vi "Destroy.vi"(0 "reference":refnum<class "CallNode.lvclass">, 5 "error in (no error)":errorcluster) -> (15 "# of objects":i32, 19 "error out":errorcluster)   [LabVIEW 2014, in "CallNode.lvclass"]
doc: "Destroys a CallNode object created with a CallNode constructor VI.\n\n[GOOP 2.3]"
uses:
  <resource>/Framework/Providers/Open_GDS/UML/CallNode_class/CallNode.lvclass
  <resource>/Framework/Providers/Open_GDS/UML/RectangularNode_class/RectangularNode.lvclass
panel:
  out "reference out":refnum<class "CallNode.lvclass">
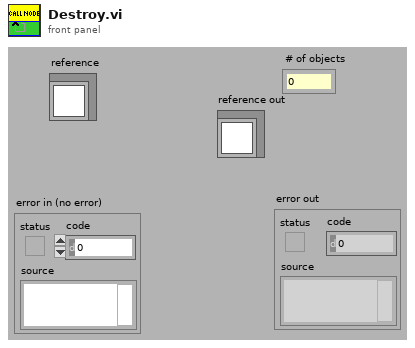
[diagram p1: front panel]
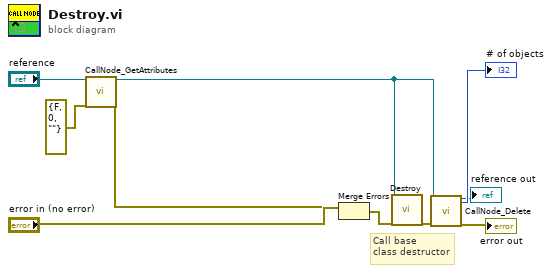
[diagram p0: block diagram]
diagram:
  # "Call base\nclass destructor"
  n1 = call <resource>:"CallNode_GetAttributes.vi"("reference in"="reference", "error in (no error)"=errorcluster {"status"=FALSE, "code"=0, "source"=""}) -> ("reference out"=w2:refnum<class "CallNode.lvclass">, "error out"=w5:errorcluster)  [unwired: 16 out]
  n2 = Merge Errors("error in (no error)", w5) -> (w3:errorcluster)
  n3 = call-parent "Destroy.vi"("reference"=w2, "error in (no error)"=w3) -> ("error out"=w1:errorcluster)  [unwired: 16 in, 1 out]
  n4 = call <resource>:"CallNode_Delete.vi"("reference in"=w2, "error in (no error)"=w1) -> ("reference out"=→"reference out":refnum<class "CallNode.lvclass">, "# of objects"=→"# of objects":i32, "error out"=→"error out":errorcluster)  [unwired: 15 out]
